vi "set_settings_cluster.vi"(8 "error in (no error)":errorcluster, 10 "settings cluster in":variant, 11 "ScanHeadDL090202 in":refnum<class "ScanHeadDL090202.lvclass">) -> (0 "error out":errorcluster, 3 "ScanHeadDL090202 out":refnum<class "ScanHeadDL090202.lvclass">)   [LabVIEW 2010, in "ScanHeadDL090202.lvclass"]
uses:
  ScanHeadDL090202.lvclass
  ScanHeadDL090202.lvclass/ScanHeadDL090202.ctl
  common/classes/ErrorController/ErrorController/class_data.vi
  common/classes/ErrorController/ErrorController/ErrorController.lvclass
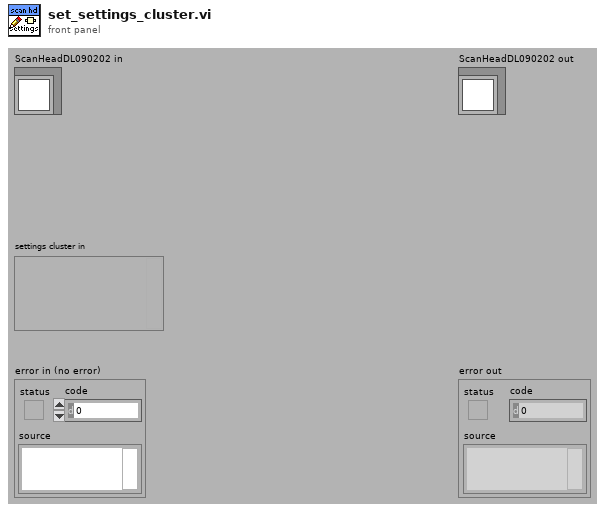
[diagram p1: front panel]
types:
  T1 = typedef "ScanHeadDL090202.lvclass/settings_cluster.ctl" = cluster{"Zoom":dbl, "Intensity":dbl, "AngleZ":dbl[unit], "AngleX":dbl[unit], "OffsetX":dbl[unit], "OffsetY":dbl[unit], "OffsetZ":dbl[unit], "ScatteringLength":dbl[unit], "ScannerDelayX":i32, "ScannerDelayY":i32, "ScannerDelayZ":i32}
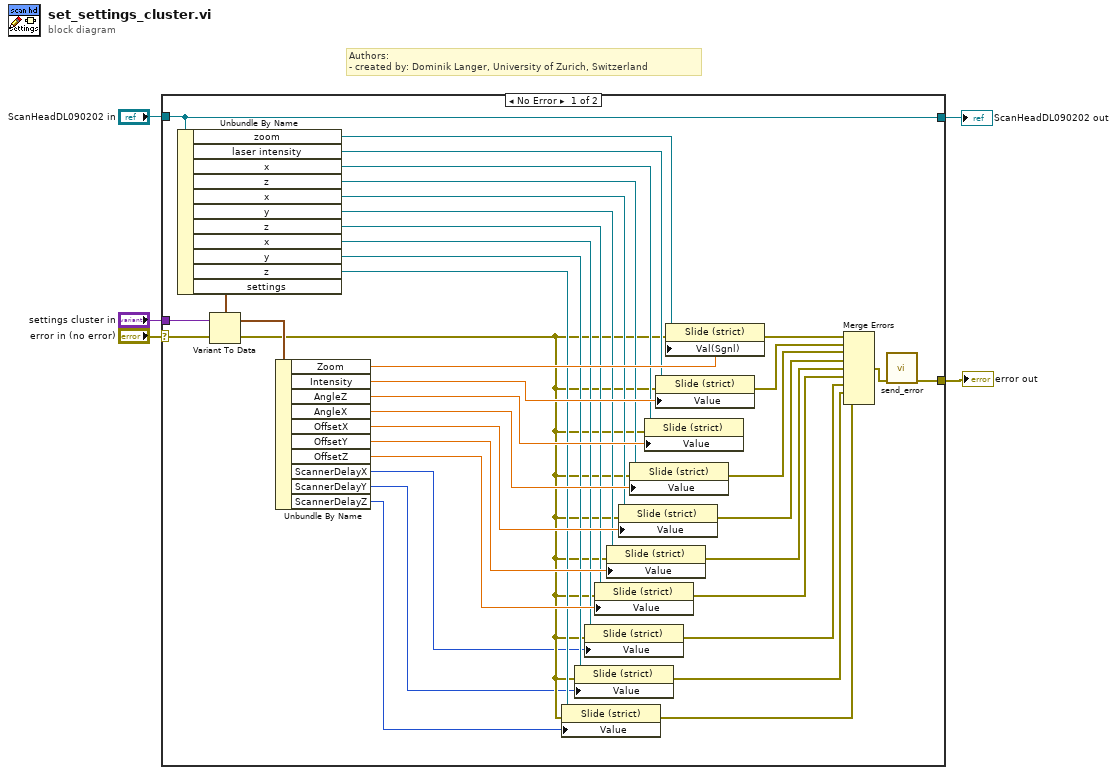
[diagram p0: block diagram]
diagram:
  # "Authors: \n- created by: Dominik Langer, University of Zurich, Switzerland"
  n1 = case shown="No Error" "error in (no error)" {
    selector: "error in (no error)" -> [w8 w43]
    tunnel: "ScanHeadDL090202 in" -> [w6 w44]
    tunnel: [w16 w43] -> w3
    tunnel: [w6 w44] -> w2
    tunnel: "settings cluster in" -> [w7 _]
    frame No Error {
      n2 = Unbundle By Name(w6) -> ("zoom"=w41:refnum<vi>, "laser intensity"=w39:refnum<vi>, "x"=w36:refnum<vi>, "z"=w35:refnum<vi>, "x"=w33:refnum<vi>, "y"=w29:refnum<vi>, "z"=w28:refnum<vi>, "x"=w26:refnum<vi>, "y"=w25:refnum<vi>, "z"=w24:refnum<vi>, "settings"=w9:T1)
      n3 = Variant To Data(error in=w8, Variant=w7, type=w9) -> (error out=w23:errorcluster, data=w42:T1)
      n4 = Unbundle By Name(w42) -> ("Zoom"=w40:dbl, "Intensity"=w38:dbl, "AngleZ"=w37:dbl[unit], "AngleX"=w34:dbl[unit], "OffsetX"=w32:dbl[unit], "OffsetY"=w31:dbl[unit], "OffsetZ"=w30:dbl[unit], "ScannerDelayX"=w22:i32, "ScannerDelayY"=w21:i32, "ScannerDelayZ"=w20:i32)
      n5 = property class="Slide (strict)"(reference=w24, error in=w23, "Value"=w20) -> (error out=w10:errorcluster)  [unwired: 1 out]
      n6 = property class="Slide (strict)"(reference=w25, error in=w23, "Value"=w21) -> (error out=w11:errorcluster)  [unwired: 1 out]
      n7 = property class="Slide (strict)"(reference=w26, error in=w23, "Value"=w22) -> (error out=w12:errorcluster)  [unwired: 1 out]
      n8 = property class="Slide (strict)"(reference=w28, error in=w23, "Value"=w30) -> (error out=w13:errorcluster)  [unwired: 1 out]
      n9 = property class="Slide (strict)"(reference=w29, error in=w23, "Value"=w31) -> (error out=w14:errorcluster)  [unwired: 1 out]
      n10 = property class="Slide (strict)"(reference=w33, error in=w23, "Value"=w32) -> (error out=w15:errorcluster)  [unwired: 1 out]
      n11 = property class="Slide (strict)"(reference=w35, error in=w23, "Value"=w34) -> (error out=w18:errorcluster)  [unwired: 1 out]
      n12 = property class="Slide (strict)"(reference=w36, error in=w23, "Value"=w37) -> ()  [unwired: 2 out]
      n13 = property class="Slide (strict)"(reference=w39, error in=w23, "Value"=w38) -> (error out=w19:errorcluster)  [unwired: 1 out]
      n14 = property class="Slide (strict)"(reference=w41, error in=w23, "Val(Sgnl)"=w40) -> (error out=w27:errorcluster)  [unwired: 1 out]
      n15 = Merge Errors(w27, w19, w18, w15, w14, w13, w12, w11, w10) -> (w17:errorcluster)
      n16 = call "send_error.vi"("error in (no error)"=w17) -> ("error out"=w16:errorcluster)  [unwired: 10 in]
    }
    frame Error {
    }
  }
  "error out" <- w3
  "ScanHeadDL090202 out" <- w2
